vi "Set Bias Voltage.vi"(8 "error in (no error)":errorcluster, 9 "Channel":i32, 10 "Bias Voltage (V)":dbl, 11 "Example in":refnum<class "Instrument.Framework-Template.lvclass">) -> (0 "error out":errorcluster, 3 "Example out":refnum<class "Instrument.Framework-Template.lvclass">)   [LabVIEW 2019, in "Instrument.Framework-Template.lvclass"]
uses:
  Instrument.Framework-Template.lvclass
  C:/Users/patrick/Documents/GitHub/Instrument-Framework/lvsrc/SMOs/Instrument/Instrument.lvclass
  Typedefs/Instrument.Framework-Template.Commands--Enum.ctl
  SMOs/Instrument/Instrument.lvclass/Instrument.ctl
  67792bfe-8e2c-4879-abc2-cb448bcec168.vi
  67792bfe-8e2c-4879-abc2-cb448bcec168.vi/e6734212-7c9e-4ce8-a442-683b18d6b7e6.vi
  SMOs/Instrument/API/Send and Receive.vi
  67792bfe-8e2c-4879-abc2-cb448bcec168.vi/d08038f8-4acd-46a3-976f-e1cbe8915b66.vi
  SMOs/Instrument/Private/Get Client Type.vi
  67792bfe-8e2c-4879-abc2-cb448bcec168.vi/e6734212-7c9e-4ce8-a442-683b18d6b7e6.vi/13966346-8efc-4621-92b5-7b0a79b586cf.vi
  67792bfe-8e2c-4879-abc2-cb448bcec168.vi/e6734212-7c9e-4ce8-a442-683b18d6b7e6.vi/fe0c9d59-5db3-4f69-8a14-a101932bc9c9.vi
  67792bfe-8e2c-4879-abc2-cb448bcec168.vi/d08038f8-4acd-46a3-976f-e1cbe8915b66.vi/f511e3ca-0286-475e-a7c2-1f5d487cf8b3.vi
  67792bfe-8e2c-4879-abc2-cb448bcec168.vi/d08038f8-4acd-46a3-976f-e1cbe8915b66.vi/82e5e6bd-25f6-43bf-8e4d-2f517738dcaa.vi
  67792bfe-8e2c-4879-abc2-cb448bcec168.vi/d08038f8-4acd-46a3-976f-e1cbe8915b66.vi/f511e3ca-0286-475e-a7c2-1f5d487cf8b3.vi/1a24b223-b4bf-4d15-8133-f9f08e4a3636.vi
  67792bfe-8e2c-4879-abc2-cb448bcec168.vi/d08038f8-4acd-46a3-976f-e1cbe8915b66.vi/f511e3ca-0286-475e-a7c2-1f5d487cf8b3.vi/f39604e6-85c4-4a3e-889c-dd3db40fa73a.vi
  SMOs/Instrument/Private/Get RC Connection Status.vi
  SMOs/Instrument/API/Enum to String.vi
  SMOs/RemoteControl/API/Send and Receive.vi
  <vilib>/Utility/Data Type/Get Type Information.vi
  <vilib>/JDP Science/JSONtext/JSON text to Variant.vi
  SMOs/Instrument/API/Instrument.GetPublicEvents.vi
  <vilib>/JDP Science/JSONtext/Variant to JSON Text.vi
  <vilib>/National Instruments/GUID Generator/Guid Generator.vi
  SMOs/Instrument/API/Instrument.MessageToProcess.vi
  SMOs/Instrument/Private/Instrument.MessageFromProcess.EventStructure.vi
  <vilib>/JDP Science/JSONtext/LVClass Serializer/JSONtext LVClass Serializer.lvclass
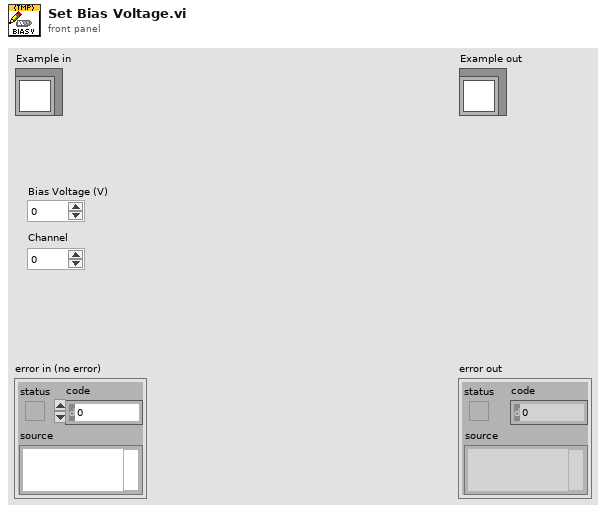
[diagram p1: front panel]
types:
  T1 = typedef "Instrument.Framework-Template.lvclass/Instrument.Framework-Template.Commands--Enum.ctl" = enum16{"command0", "command1", "command2"}
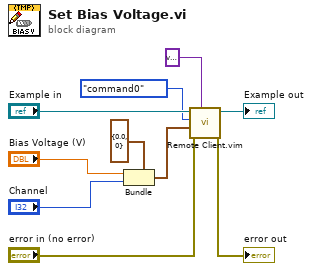
[diagram p0: block diagram]
diagram:
  n1 = Bundle(cluster=cluster{"Bias Voltage (V)":dbl, "Channel":i32} {"Bias Voltage (V)"=0.0, "Channel"=0} ("output cluster"), "Bias Voltage (V)"="Bias Voltage (V)", "Channel"="Channel") -> (w3:cluster{"Bias Voltage (V)":dbl, "Channel":i32})
  n2 = call "Remote Client.vim"("Data Out type"=variant, "error in (no error)"="error in (no error)", "params"=w3, "method"=Instrument.Framework-Template.Commands--Enum."command0" ("Commands"), "Instrument in"="Example in") -> ("error out"=→"error out":errorcluster, "Instrument out"=→"Example out":refnum<class "Instrument.Framework-Template.lvclass">)  [unwired: 3 in, 2 out]
